vi "9093_第8回課題_山口修平.vi"() -> ()   [LabVIEW 2020]
panel:
  in  "振幅[V] 2":dbl(slide) scale=0.0..10.0
  in  "周波数[kHz] 2":dbl(slide) scale=0.0..10.0
  in  "ノイズレベル[V] 2":dbl(knob) scale=0.0..1.0
  out "信号波":dynamicdata(graph)
  in  "停止":bool
  in  "振幅[V]":dbl(slide) scale=0.0..20.0
  in  "周波数[kHz]":dbl(slide) scale=0.0..100.0
  in  "ノイズレベル[V]":dbl(knob) scale=0.0..1.0
  out "搬送波":dynamicdata(graph)
  in  "トリガ 2":bool
  in  "トリガ":bool
  out "合成波":dynamicdata(graph)
  out "フィルタ":dynamicdata(graph)
  in  "Lower Cut-Off":dbl=100.0 caption="低域カットオフ周波数"
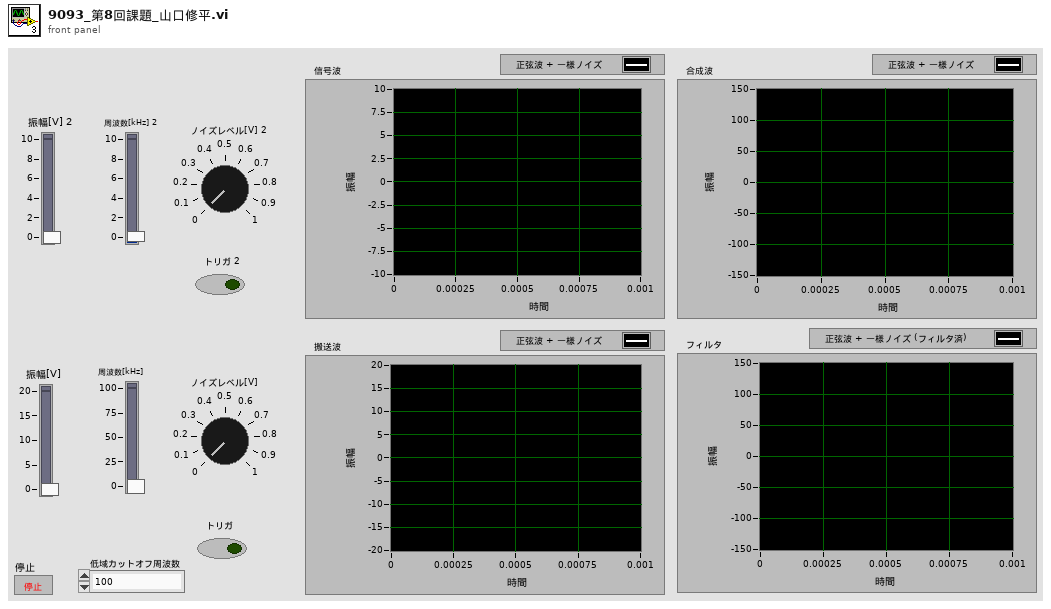
[diagram p1: front panel]
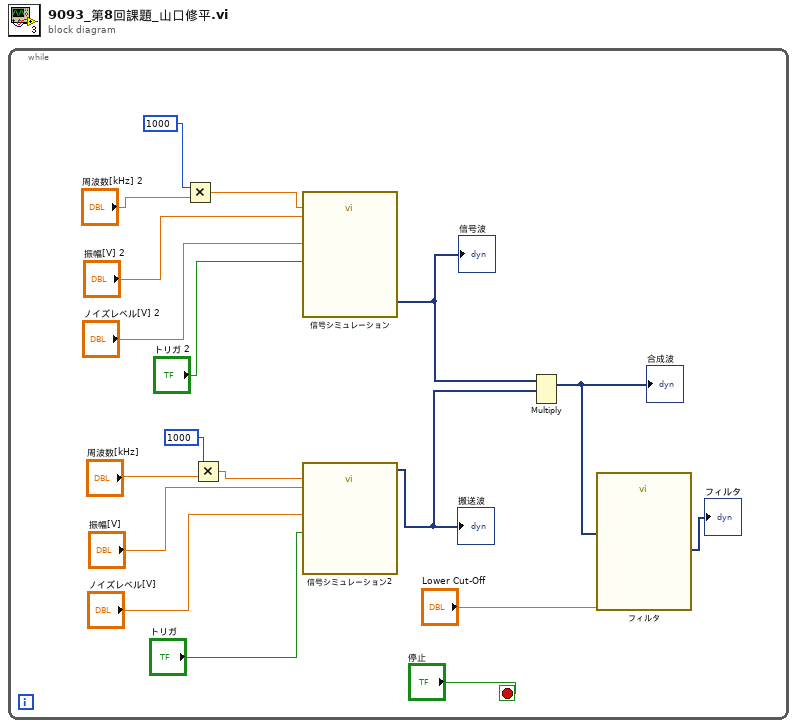
[diagram p0: block diagram]
diagram:
  n1 = while {
    stop <- "停止" stop-if-true
    n2 = Multiply(x=1000, y="周波数[kHz] 2") -> (x*y=w10:dbl)
    n3 = Multiply(x=1000, y="周波数[kHz]") -> (x*y=w7:dbl)
    n4 = call "信号シミュレーション"("Reset Signal"="トリガ 2", "Frequency"=w10, "Amplitude"="振幅[V] 2", "ノイズ振幅"="ノイズレベル[V] 2") -> ("正弦波 と 一様ノイズ"=w5:dynamicdata)  [unwired: 10 in, 1 out]
    "信号波" <- w5
    n5 = call "信号シミュレーション2"("Reset Signal"="トリガ", "Frequency"=w7, "Amplitude"="振幅[V]", "ノイズ振幅"="ノイズレベル[V]") -> ("正弦波 と 一様ノイズ"=w4:dynamicdata)  [unwired: 10 in, 1 out]
    "搬送波" <- w4
    n6 = Multiply(1:w4, 2:w5) -> (0:w1:dynamicdata)  [unwired: 1 in, 1 out]
    "合成波" <- w1
    n7 = call "フィルタ"("Lower Cut-Off"="Lower Cut-Off", "Signal"=w1) -> ("Filtered Signal"=→"フィルタ":dynamicdata)  [unwired: 8 in, 1 out]
  }
